vi "BooleanCommand_Example.vi"() -> ()   [LabVIEW 2019]
uses:
  <vilib>/Rock Robotics/WPI/ThirdParty/JAS_Junk/TrajLib/Trajectory_Library.lvlib
  <vilib>/Rock Robotics/WPI/ThirdParty/JAS_Junk/TrajLib/Enum/AutoHelperSequence_Step_Enum.ctl
panel:
  out "Auto Step Number":T1
  out "Auto\nActive":bool
  in  "Start\nAutonomous":bool
  in  "Teleop\nAction 1":bool
  in  "Teleop\nAction 2":bool
  out "Action Two":bool
  out "Waveform Chart":cluster{i16, i16}(graph)
  out "Action-One":bool
  # "BOOLEAN COMMAND EXAMPLE"
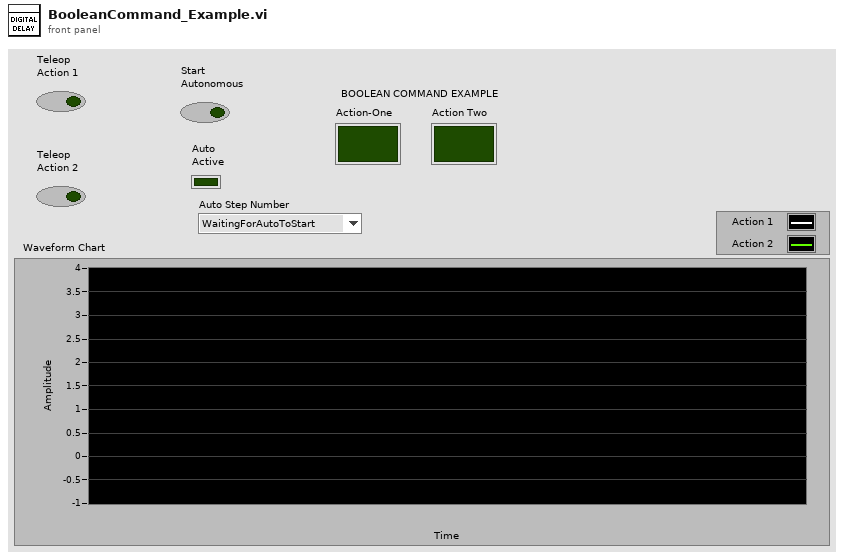
[diagram p1: front panel]
types:
  T1 = typedef "Trajectory_Library.lvlib/AutoHelperSequence_Step_Enum.ctl" = enum16{"WaitingForAutoToStart", "Step 1", "Step 2", "Step 3", "Step 4", "Step 5", "Step 6", "Step 7", "Step 8", "Step 9", "Step 10", "Step 11", "Step 12", "Step 13", "Step 14", "Step 15", "Step 16", "Step 17", "Step 18", "Step 19", "Step 20", "Step 21", "Step 22", "Step 23", "Step 24", "Step 25", "Step 26", "Step 27", "Step 28", "Step 29", "Step 30", "Step 31", "Step 32", "AutoDone"}
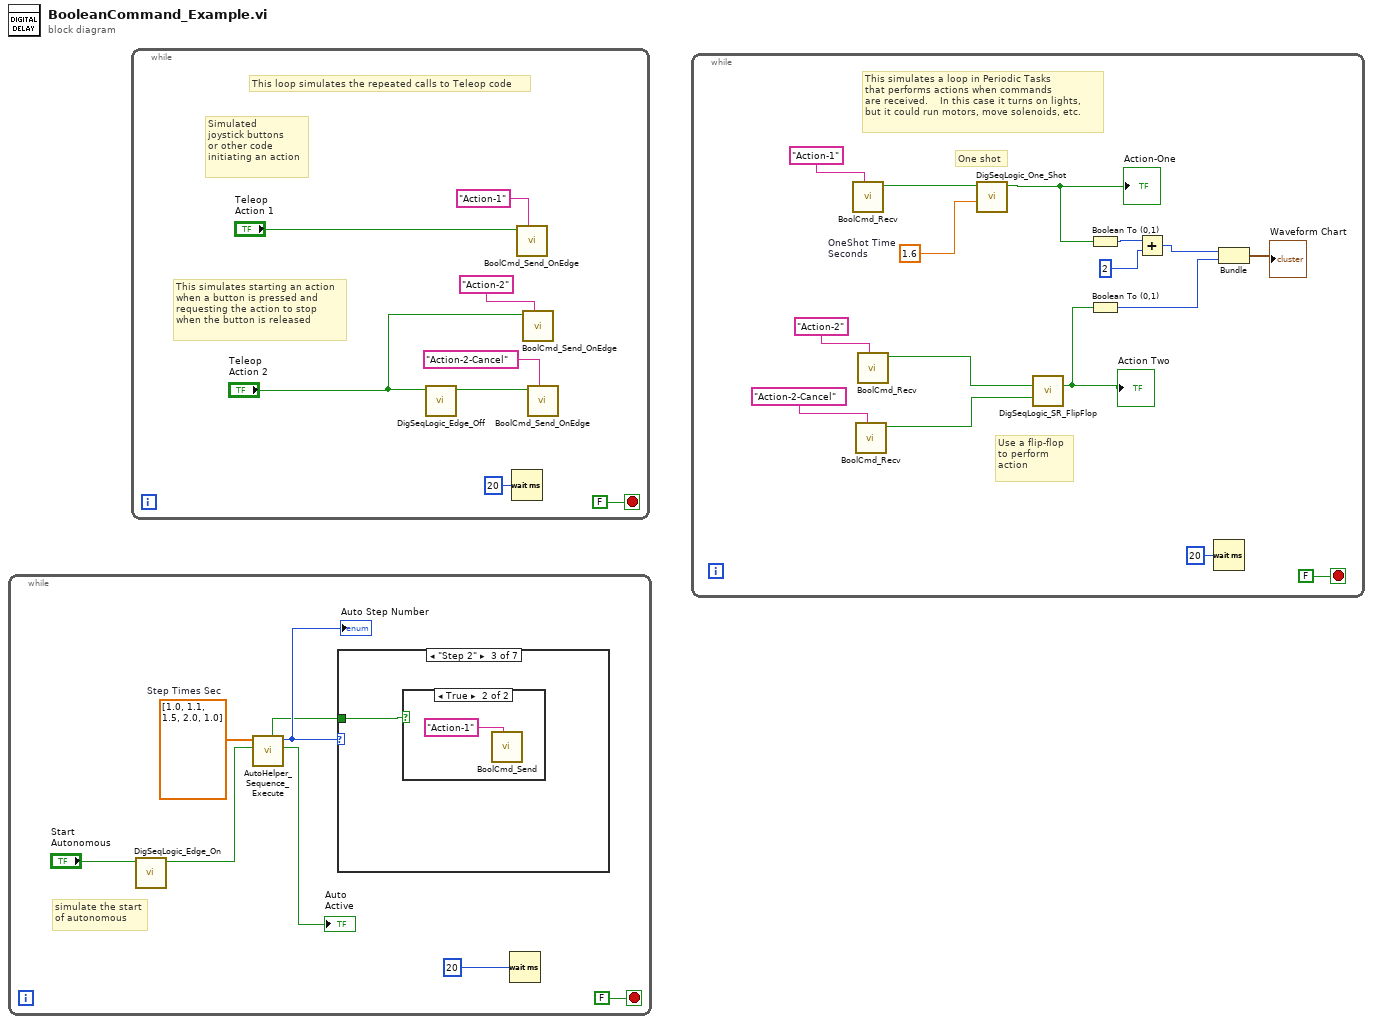
[diagram p0: block diagram]
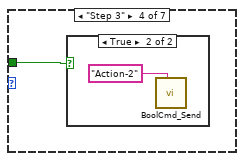
[diagram p5: hidden frame]
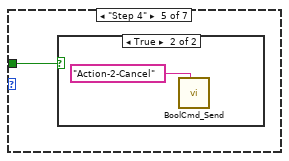
[diagram p7: hidden frame]
diagram:
  n1 = while {
    stop <- FALSE stop-if-true
    w5 = dbl[] [1.0, 1.1, 1.5, 2.0, 1.0]  # Step Times Sec
    # "simulate the start\nof autonomous"
    n2 = call <vilib>:"DigSeqLogic_Edge_On.vi"("Input"="Start\nAutonomous") -> ("On Edge"=w4:bool)  [unwired: 10 in]
    n3 = call <vilib>:"AutoHelper_Sequence_Execute.vi"("Initiate"=w4, "Step Times Sec"=w5) -> ("Seq  Active"=→"Auto\nActive":bool, "Step Number State"=w3:T1, "New Step"=w2:bool)  [unwired: 5 in, 2 out]
    "Auto Step Number" <- w3
    n4 = case shown="\"Step 2\"" w3 {
      tunnel: w2 -> [_ _ w9 w11 w13 _ _]
      frame "WaitingForAutoToStart", Default {
      }
      frame "Step 1" {
        # "do nothing"
      }
      frame "Step 2" {
        n5 = case shown="True" w9 {
          frame False {
          }
          frame True {
            n6 = call <vilib>:"BoolCmd_Send.vi"("Command Name"="Action-1") -> ()  [unwired: 10 in, 1 out]
          }
        }
      }
      frame "Step 3" {
        n7 = case shown="True" w11 {
          frame False {
          }
          frame True {
            n8 = call <vilib>:"BoolCmd_Send.vi"("Command Name"="Action-2") -> ()  [unwired: 10 in, 1 out]
          }
        }
      }
      frame "Step 4" {
        n9 = case shown="True" w13 {
          frame False {
          }
          frame True {
            n10 = call <vilib>:"BoolCmd_Send.vi"("Command Name"="Action-2-Cancel") -> ()  [unwired: 10 in, 1 out]
          }
        }
      }
      frame "Step 5" {
      }
      frame "AutoDone" {
      }
    }
    n11 = Wait (ms)(milliseconds to wait=u32 20 ("milliseconds to wait 2")) -> ()  [unwired: 1 out]
  }
  n12 = while {
    stop <- FALSE stop-if-true
    # "This simulates starting an action\nwhen a button is pressed and\nrequesting the action to stop\nwhen the button is released"
    # "Simulated\njoystick buttons\nor other code \ninitiating an action"
    # "This loop simulates the repeated calls to Teleop code"
    n13 = call <vilib>:"DigSeqLogic_Edge_Off.vi"("Input"="Teleop\nAction 2") -> ("Off Edge"=w16:bool)  [unwired: 10 in]
    n14 = Wait (ms)(milliseconds to wait=u32 20) -> ()  [unwired: 1 out]
    n15 = call <vilib>:"BoolCmd_Send_OnEdge.vi"("Command Name"="Action-1", "Value"="Teleop\nAction 1") -> ()  [unwired: 9 in, 1 out]
    n16 = call <vilib>:"BoolCmd_Send_OnEdge.vi"("Command Name"="Action-2", "Value"="Teleop\nAction 2") -> ()  [unwired: 9 in, 1 out]
    n17 = call <vilib>:"BoolCmd_Send_OnEdge.vi"("Command Name"="Action-2-Cancel", "Value"=w16) -> ()  [unwired: 9 in, 1 out]
  }
  n18 = while {
    stop <- FALSE stop-if-true
    w25 = 1.6  # OneShot Time Seconds
    # "One shot"
    # "Use a flip-flop\nto perform\naction"
    # "This simulates a loop in Periodic Tasks\nthat performs actions when commands\nare received.    In this case it turns on lights,\nbut it could run motors, move solenoids, etc."
    n19 = call <vilib>:"BoolCmd_Recv.vi"("Command Name"="Action-1") -> ("New Request"=w24:bool)  [unwired: 9 in, 1 out]
    n20 = call <vilib>:"BoolCmd_Recv.vi"("Command Name"="Action-2-Cancel") -> ("New Request"=w27:bool)  [unwired: 9 in, 1 out]
    n21 = call <vilib>:"BoolCmd_Recv.vi"("Command Name"="Action-2") -> ("New Request"=w28:bool)  [unwired: 9 in, 1 out]
    n22 = call <vilib>:"DigSeqLogic_One_Shot.vi"("OneShot"=w25, "Input"=w24) -> ("Output"=w23:bool)  [unwired: 8 in, 1 out]
    "Action-One" <- w23
    n23 = call <vilib>:"DigSeqLogic_SR_FlipFlop.vi"("Set"=w28, "Reset"=w27) -> ("Output"=w26:bool)  [unwired: 12 in, 1 out]
    "Action Two" <- w26
    n24 = Boolean To (0,1)(Boolean=w23) -> (0, 1=w34:i16)
    n25 = Boolean To (0,1)(Boolean=w26) -> (0, 1=w32:i16)
    n26 = Add(x=w34, y=i16 2) -> (x+y=w33:i16)
    n27 = Wait (ms)(milliseconds to wait=u32 20) -> ()  [unwired: 1 out]
    n28 = Bundle(w33, w32) -> (→"Waveform Chart":cluster{i16, i16})  [unwired: 1 in]
  }
